vi "Write Export Operation Errors.vi"(8 "Error In":errorcluster, 10 "Export Operation Errors":errorcluster, 11 "Export in":refnum<class "Export.lvclass">) -> (0 "Error Out":errorcluster, 3 "Export out":refnum<class "Export.lvclass">)   [LabVIEW 2017, in "CL_G3_VIComponentBuilder.lvlib" / "Export.lvclass"]
uses:
  Export.lvclass
  Export.lvclass/Export.ctl
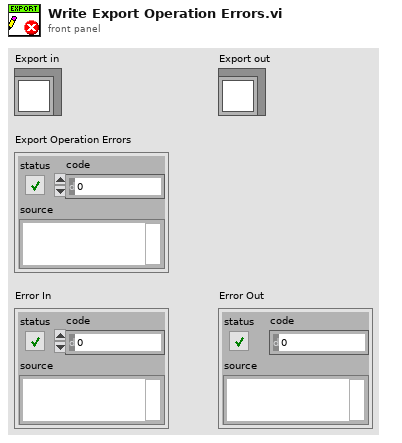
[diagram p1: front panel]
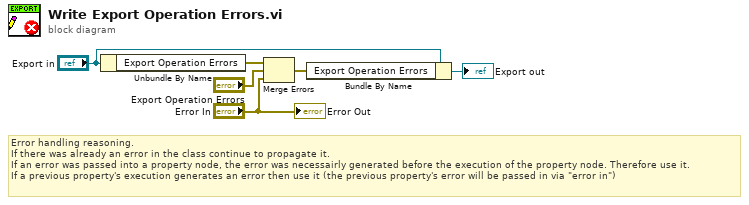
[diagram p0: block diagram]
diagram:
  # "Error handling reasoning.\nIf there was already an error in the class continue to propagate it.\nIf an error was passed into a property node, the error was necessairly generated before the execution of the property node. Therefore use it.\nIf a previous property's execution generates an error then use it (the previous property's error will be passed in via \"error in\")"
  n1 = Unbundle By Name("Export in") -> ("Export Operation Errors"=w3:errorcluster)
  n2 = Merge Errors(w3, "Export Operation Errors", "Error In") -> (w2:errorcluster)
  n3 = Bundle By Name(cluster="Export in", "Export Operation Errors"=w2) -> (→"Export out":refnum<class "Export.lvclass">)
  "Error Out" <- "Error In"
